vi "Flat Secuence bloqueante.vi"() -> ()   [LabVIEW 2020]
panel:
  out "Boolean 2":bool
  in  "Boolean":bool
  out "Thermometer":u32(slide) scale=0.0..100.0
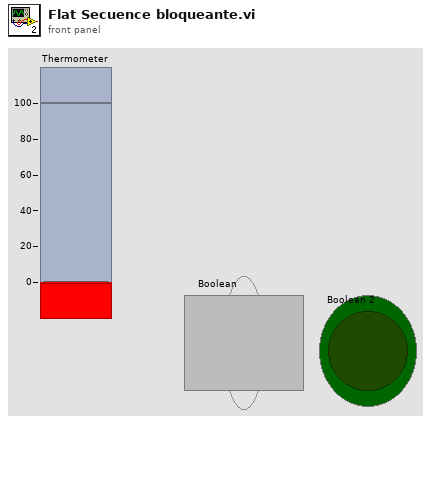
[diagram p1: front panel]
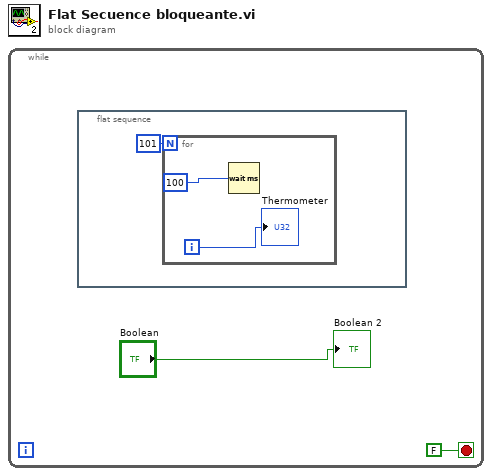
[diagram p0: block diagram]
diagram:
  n1 = while {
    stop <- FALSE stop-if-true
    n2 = flat-sequence {
      frame #0 {
        n3 = for {
          N: 101 -> [_]
          i -> [w5]
          n4 = Wait (ms)(milliseconds to wait=u32 100) -> ()  [unwired: 1 out]
          "Thermometer" <- w5
        }
      }
    }
    "Boolean 2" <- "Boolean"
  }
